vi "agilent_test_2.vi"() -> ()   [LabVIEW 2016]
uses:
  <vilib>/Instr/_visa.llb/VISA Open Access Mode.ctl
panel:
  out "VISA resource name out":refnum<visa-resource-name>
  out "error out":errorcluster
  out "read buffer":string
  in  "VISA resource name":refnum<visa-resource-name>="vna"
  in  "error in (no error)":errorcluster
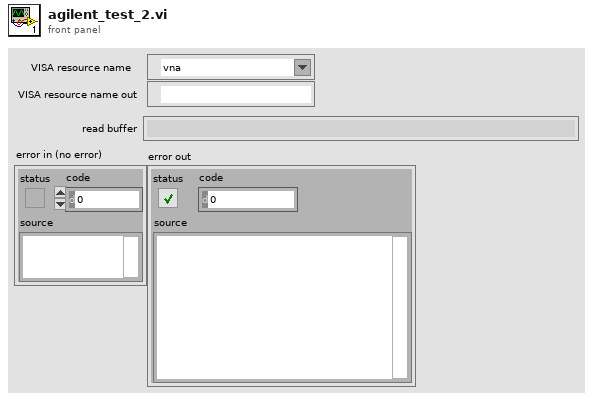
[diagram p1: front panel]
types:
  T1 = typedef "VISA Open Access Mode.ctl" = u32
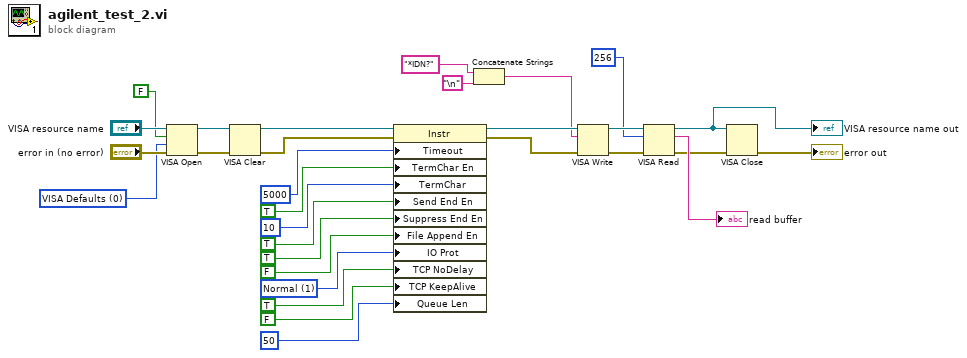
[diagram p0: block diagram]
diagram:
  w4 = T1 0 items=["VISA Defaults"=0, "Exclusive Lock"=1, "Load Configured Settings"=4] ("Access Mode")
  w18 = u16 1 items=["Normal"=1, "VXI/FDC"=2, "GPIB/HS488"=3, "Serial-TCPIP-USB/488 Strings"=4, "USBTMC/Vendor-Specific"=5] ("Message Based Settings:IO Protocol")
  n1 = VISA Open(duplicate session (F)=FALSE, access mode=w4, error in (no error)="error in (no error)", VISA resource name="VISA resource name") -> (VISA resource name=w28:refnum<visa-resource-name>, error out=w27:errorcluster)  [unwired: 1 in]
  n2 = VISA Clear(VISA resource name=w28, error in (no error)=w27) -> (VISA resource name out=w26:refnum<visa-resource-name>, error out=w25:errorcluster)
  n3 = property class="Instr"(reference=w26, error in=w25, "Timeout"=u32 5000 ("General Settings:Timeout Value"), "TermChar En"=TRUE ("Message Based Settings:Termination Character Enable"), "TermChar"=u8 10 ("Message Based Settings:Termination Character"), "Send End En"=TRUE ("Message Based Settings:Send End Enable"), "Suppress End En"=TRUE ("Message Based Settings:Suppress End Enable"), "File Append En"=FALSE ("Message Based Settings:File Append Enable"), "IO Prot"=w18, "TCP NoDelay"=TRUE ("TCP/IP Settings:No Packet Delay"), "TCP KeepAlive"=FALSE ("TCP/IP Settings:Keep-Alive Packets"), "Queue Len"=u32 50 ("General Settings:Maximum Queue Length")) -> (reference out=w13:refnum<visa-resource-name>, error out=w14:errorcluster)
  n4 = Concatenate Strings("*IDN?" ("string"), "\n") -> (w8:string)
  n5 = VISA Write(VISA resource name=w13, write buffer=w8, error in (no error)=w14) -> (VISA resource name out=w12:refnum<visa-resource-name>, error out=w11:errorcluster)  [unwired: 1 out]
  n6 = VISA Read(VISA resource name=w12, byte count=u32 256, error in (no error)=w11) -> (VISA resource name out=w2:refnum<visa-resource-name>, read buffer=→"read buffer":string, error out=w3:errorcluster)  [unwired: 1 out]
  "VISA resource name out" <- w2
  n7 = VISA Close(VISA resource name=w2, error in (no error)=w3) -> (error out=→"error out":errorcluster)
